vi "RSZVB RF Source Calibration.vi"(8 "error in (no error)":errorcluster {"code" format="%.0x"}, 10 "Channel (1)":i32=1, 11 "VISA session":refnum<visa-resource-name>) -> (0 "error out":errorcluster {"code" format="%.0x"}, 3 "dup VISA session":refnum<visa-resource-name>)   [LabVIEW 2011]
doc: "This VI starts the RF source calibration (1st power calibration step for mixer measurements), stores and applies the calibration data.\n\nNote(s):\n\n(1) For some measurements the default set timeout can be insufficient. To set higher timeout use VI RSZVB Set Time Out.vi.\n\nRemote-control command(s):\nSOURce<Ch>:POWer<Pt>:CORRection:MIXer:RF[:ACQuire]"
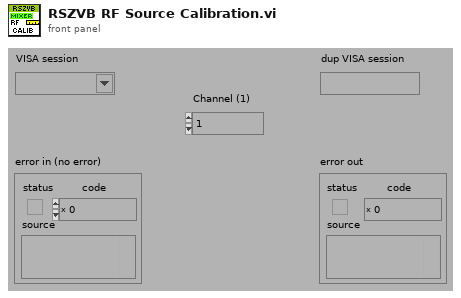
[diagram p1: front panel]
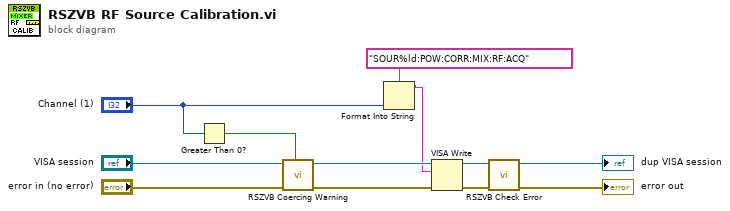
[diagram p0: block diagram]
diagram:
  n1 = Greater Than 0?(x="Channel (1)") -> (x > 0?=w6:bool)
  n2 = call "RSZVB Coercing Warning.vi"("In Range?"=w6, "error in (no error)"="error in (no error)", "VISA session"="VISA session") -> ("error out"=w11:errorcluster, "dup VISA session"=w12:refnum<visa-resource-name>)  [unwired: 7 in]
  n3 = Format Into String(format string="SOUR%ld:POW:CORR:MIX:RF:ACQ", "Channel (1)") -> (resulting string=w7:string)  [unwired: 2 in, 1 out]
  n4 = VISA Write(VISA resource name=w12, write buffer=w7, error in (no error)=w11) -> (VISA resource name out=w9:refnum<visa-resource-name>, error out=w10:errorcluster)  [unwired: 1 out]
  n5 = call "RSZVB Check Error.vi"("error in (no error)"=w10, "VISA session"=w9) -> ("error out"=→"error out":errorcluster, "dup VISA session"=→"dup VISA session":refnum<visa-resource-name>)  [unwired: 8 in]
